vi "Create Plugin Section.vi"(7 "GUID (Default Section)":string="03D3BB89-1485-13A6-56005DE6430FF8B7", 8 "error in (no error)":errorcluster, 10 "Plugin Configurations":refnum<class "Plugin Configuration.lvclass">[](array[class]), 11 "Item Ref in":T1 format="%.0x") -> (0 "error out":errorcluster, 2 "Plugin Section refs":T1[](array[typedef]) format="%.0x", 3 "Item Ref out":T1 format="%.0x")   [LabVIEW 2017, in "DSF System Explorer.lvlib"]
uses:
  DSF System Explorer.lvlib
  <vilib>/NI Veristand/Custom Device API/Custom Device Item Ref.ctl
  DSF Core.lvlibp/Classes/Configuration/Base/Plugin/Plugin Configuration.lvclass
  <vilib>/NI Veristand/Custom Device API/Custom Device API.lvlib
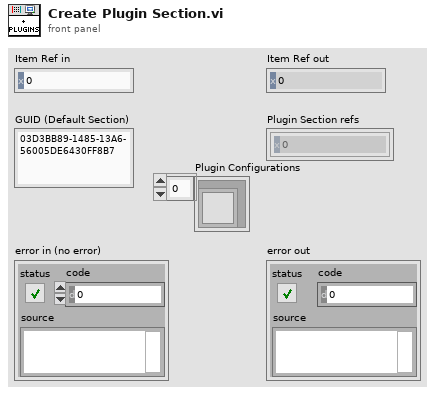
[diagram p1: front panel]
types:
  T1 = typedef "Custom Device API.lvlib/Custom Device Item Ref.ctl" = u64
  T2 = typedef "DSF Core.lvlibp/DSF Core Plugin Configuration.ctl" = cluster{"name":string, "components":string[], "cycle timing":T3}
  T3 = typedef "DSF Core.lvlibp/DSF Timing Info.ctl" = cluster{"priority":u64, "decimation":u64, "offset":u64}
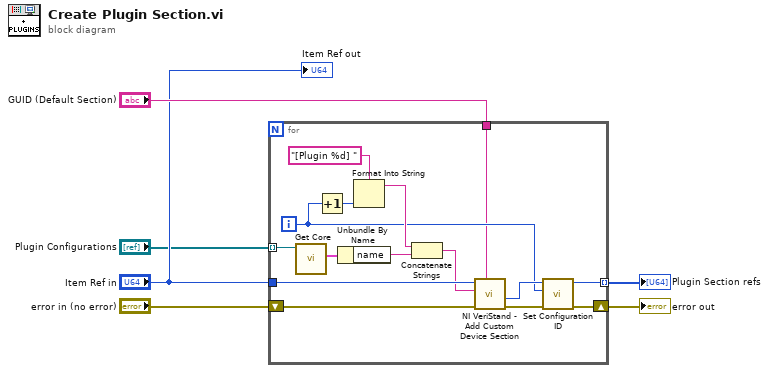
[diagram p0: block diagram]
diagram:
  n1 = for {
    tunnel: "Item Ref in" -> [w18]
    shift-right: [w14] -> w6
    shift-left: "error in (no error)" -> [w13]
    tunnel: [w15] -> w5 mode=indexing
    tunnel: "GUID (Default Section)" -> [w7]
    tunnel: "Plugin Configurations" -> [w10] mode=indexing
    i -> [w11]
    n2 = call "Get Core.vi"("Plugin Configuration in"=w10) -> ("core"=w8:T2)  [unwired: 8 in, 2 out]
    n3 = Increment(x=w11) -> (x+1=w19:i32)
    n4 = Unbundle By Name(w8) -> ("name"=w9:string)
    n5 = Format Into String(format string="[Plugin %d] ", w19) -> (resulting string=w21:string)  [unwired: 2 in, 1 out]
    n6 = Concatenate Strings(w21, w9) -> (w12:string)
    n7 = call <vilib>:"NI VeriStand - Add Custom Device Section.vi"("GUID (Default Section)"=w7, "error in (no error)"=w13, "Section Name"=w12, "Parent Ref in"=w18) -> ("error out"=w16:errorcluster, "Section Ptr"=w17:T1)  [unwired: 4 in, 2 out]
    n8 = call "Set Configuration ID.vi"("error in (no error)"=w16, "Configuration ID"=w11, "Item Ref in"=w17) -> ("error out"=w14:errorcluster, "Item Ref out"=w15:T1)  [unwired: 7 in]
  }
  "error out" <- w6
  "Plugin Section refs" <- w5
  "Item Ref out" <- "Item Ref in"
